vi "Remove Dup and Empty.vi"(11 "Array in":string[](array[string])) -> (3 "Array out":string[](array[string]))   [LabVIEW 2017]
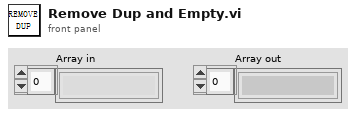
[diagram p1: front panel]
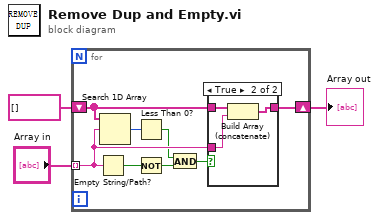
[diagram p0: block diagram]
diagram:
  n1 = for {
    tunnel: "Array in" -> [w9] mode=indexing
    shift-right: [w7] -> w1
    shift-left: string[] [] ("Array in") -> [w8]
    n2 = Empty String/Path?(string/path=w9) -> (empty?=w11:bool)
    n3 = Search 1D Array(1D array=w8, element=w9) -> (index of element=w10:i32)  [unwired: 1 in]
    n4 = Less Than 0?(x=w10) -> (x < 0?=w6:bool)
    n5 = Not(x=w11) -> (.not. x?=w5:bool)
    n6 = And(x=w6, y=w5) -> (x .and. y?=w4:bool)
    n7 = case shown="True" w4 {
      tunnel: w9 -> [_ w15]
      tunnel: w8 -> [w12 w14]
      tunnel: [w12 w13] -> w7
      frame False {
      }
      frame True {
        n8 = Build Array (concatenate)(w14, w15) -> (w13:string[])
      }
    }
  }
  "Array out" <- w1
